vi "T7MOD_Write_FLOAT32_Register.vi"(7 "FLOAT32 to Write":sgl=1.23, 8 "error in":errorcluster, 9 "LabJack FLOAT32 Register":i32=55124, 10 "Remote Port":u16=502, 11 "Remote IP Address":string="192.168.1.15") -> (0 "error out":errorcluster, 1 "Written At":timestamp)   [LabVIEW 2015]
uses:
  Serial Link Layer/NI_Modbus_Cleaned/NI Modbus121Clean.llb/MB Ethernet Master Query Write Multiple Registers (poly).vi
panel:
  # "Input"
  # "TCP Parameters"
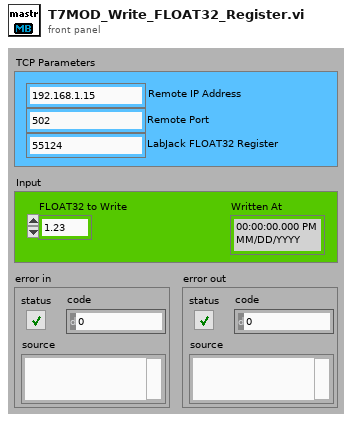
[diagram p1: front panel]
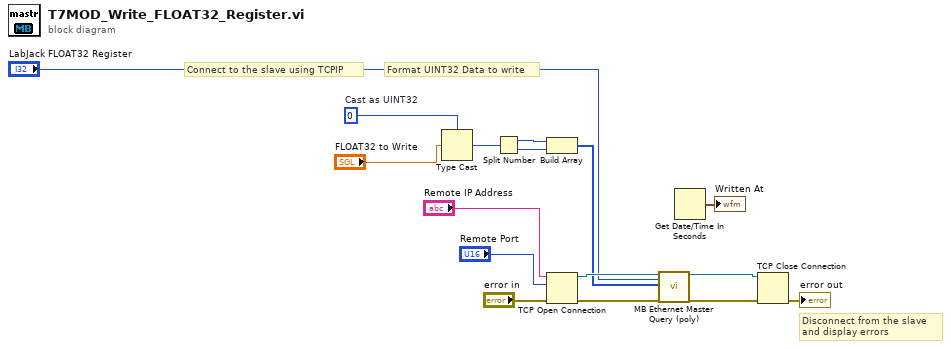
[diagram p0: block diagram]
diagram:
  w5 = u32 0  # Cast as UINT32
  # "Format UINT32 Data to write"
  # "Disconnect from the slave\nand display errors"
  # "Connect to the slave using TCPIP"
  n1 = Type Cast(type=w5, x="FLOAT32 to Write") -> (*(type *) &x=w4:u32)
  n2 = Split Number(x=w4) -> (hi(x)=w3:u16, lo(x)=w2:u16)
  n3 = Build Array(w3, w2) -> (w7:u16[])
  n4 = TCP Open Connection(address="Remote IP Address", remote port or service name="Remote Port", error in (no error)="error in") -> (connection ID=w14:refnum<k5>, error out=w13:errorcluster)  [unwired: 2 in]
  n5 = call-poly "MB Ethernet Master Query (poly).vi"("TCP Connection Refnum in"=w14, "Starting Address"="LabJack FLOAT32 Register", "Registers"=w7, "error in"=w13) -> ("TCP Connection Refnum (dup)"=w11:refnum<k5>, "error out"=w12:errorcluster)  [unwired: 13 in, 1 out]
  n6 = Get Date/Time In Seconds() -> (seconds since 1Jan1904=→"Written At":timestamp)
  n7 = TCP Close Connection(connection ID=w11, error in (no error)=w12) -> (error out=→"error out":errorcluster)  [unwired: 2 out]
